vi "Module Top Level.vi"(8 "error in (no error)":errorcluster) -> (0 "error out":errorcluster)   [LabVIEW 2018, in "File IO.lvlib"]
doc: "This is the top level VI for this module. It uses a queue for communications and is stopped user a user event. The general architecture is similar to a simple queued message handler.\n\nThe VIs associated with this module are organized in a LabVIEW Library."
uses:
  File IO.lvlib
  Private Controls/File IO Data.ctl
  Controller (Host)/Public Controls/Test Information.ctl
  Controller (Host)/Public VIs/PreorPostSB.ctl
  Controller (Host)/Public Controls/APU Select.ctl
  Top Level/Shared Controls/Analyzed Data Sets.ctl
  Top Level/Shared Controls/All Data Cluster.ctl
  Top Level/Shared Controls/Acq Data.ctl
  Top Level/Shared Controls/APU Setup File.ctl
  <vilib>/Utility/NIReport.llb/NI_report.lvclass
  Private Controls/Module Data.ctl
  Private Controls/Module Action.ctl
  Public Controls/Write to Report.ctl
  Public Controls/Report Sheet Names.ctl
  <vilib>/Utility/NIReport.llb/Report Type.ctl
  Public Controls/Variables.ctl
  Testing UI 3/Public Controls/Accel Config.ctl
  Testing UI 3/Private Controls/Cutoff Frequency.ctl
  <vilib>/Utility/file.llb/Write Delimited Spreadsheet (string).vi
  Error Handler/Error Handler.lvlib
  Controller (Host)/Controller (Host).lvlib
  Testing UI 1/Testing UI 1.lvlib
  Testing UI 2/Testing UI 2.lvlib
  Testing UI 3/Testing UI 3.lvlib
  <vilib>/Utility/NIReport.llb/NI_ReportGenerationCore.lvlib
panel:
  in  "Record Data Test":bool
  in  "Test APU RUN TIME LOG":bool
  # "File I/O"
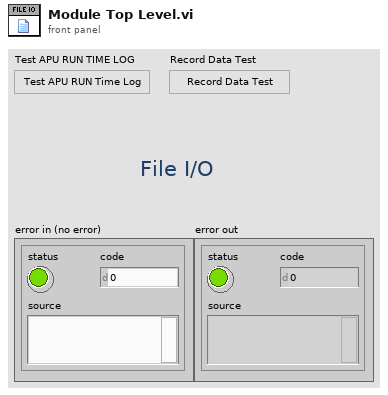
[diagram p1: front panel]
types:
  T1 = typedef "File IO.lvlib/File IO Data.ctl" = cluster{"System Log File":path, "Data File":path, "Work Order Folder":path, "Report Template Folder":path, "Report Folder":path, "Report File":path, "APU Setup Folder":path, "Testing State":bool, "Recording State":bool, "Test Information":T2, "Crash Log Data":T5, "Group Name":string, "APU Setup":T8, "ChannelTagsToLog":string[], "report ref":refnum<class "NI_report.lvclass">, "APU Setup File":path, "RunTimes":string[], "ReportHeader":string[]}
  T2 = typedef "Controller (Host).lvlib/Test Information.ctl" = cluster{"APU Part Number:":string, "Model:":string, "Serial Number:":string, "Customer:":string, "Work Order:":string, "Pre or Post SB":T3, "Run Count":i32, "APU Selected":T4}
  T3 = typedef "Controller (Host).lvlib/PreorPostSB.ctl" = string
  T4 = typedef "Controller (Host).lvlib/APU Select.ctl" = string
  T5 = typedef "Analyzed Data Sets.ctl" = T6[]
  T6 = typedef "All Data Cluster.ctl" = cluster{"AI":T7, "Accel Data":cluster{"Accel RMS(in/sec2)":dbl[], "Accel Peak(in/sec2)":dbl[], "Velocity RMS(in/sec)":dbl[], "Velocity Peak(in/sec)":dbl[]}, "Temps":cluster{"01-00-9213":dbl[], "01-01-9213":dbl[], "01-02-9213":dbl[]}, "00-03-9402(RPM)":dbl[], "02-04-9871":dbl[], "ARINC":sgl[]}
  T7 = typedef "Acq Data.ctl" = cluster{"00-00-9220":dbl[], "00-01-9220":dbl[], "02-02-9219":dbl[], "02-03-9227":dbl[], "02-05-9205":dbl[]}
  T8 = typedef "APU Setup File.ctl" = cluster{"Sensor Info":string[][], "Variables":string[][], "CMM Table 106":string[][], "CMM Table 106B ":string[][], "Accel Config":string[][], "Report Sheet 1":string[][], "Report Sheet 2":string[][], "Report Sheet 3":string[][]}
  T9 = typedef "File IO.lvlib/Write to Report.ctl" = cluster{"Sheet Name":T10, "Cell #":string, "Data":string}
  T10 = typedef "File IO.lvlib/Report Sheet Names.ctl" = string
  T11 = typedef "NI_ReportGenerationCore.lvlib/Report Type.ctl" = enum16{"HTML", "Word", "Excel"}
  T12 = enum16{"maximized", "minimized", "normal", "no change"}
  T13 = typedef "File IO.lvlib/Variables.ctl" = cluster{"AIN":dbl, "SG60":dbl, "K":dbl, "OrifDia":dbl, "FuelPressure":dbl}
  T14 = typedef "Testing UI 3.lvlib/Accel Config.ctl" = cluster{"PS Sens":dbl, "GB Sens":dbl, "FAN Sens":dbl, "PS Cutoff Frequency":T15, "GB Cutoff Frequency":T15, "Fan Cutoff Frequency":T15}
  T15 = typedef "Testing UI 3.lvlib/Cutoff Frequency.ctl" = cluster{"LP Passband":dbl, "HP Stopband":dbl, "LP Stopband":dbl, "HP Passband":dbl}
  T16 = typedef "File IO.lvlib/Module Data.ctl" = cluster{"Data":variant, "Action":T17}
  T17 = typedef "File IO.lvlib/Module Action.ctl" = enum8{"Timeout", "OpenReport", "Continue Test", "Init", "Error", "Exit", "Save Accel Data", "Set Recording State", "Log APU RunTime", "Start New Test", "Create New Reports", "Write to System Log", "Save Variables", "Load APU Setup File", "Increment Run Count", "Write To Report"}
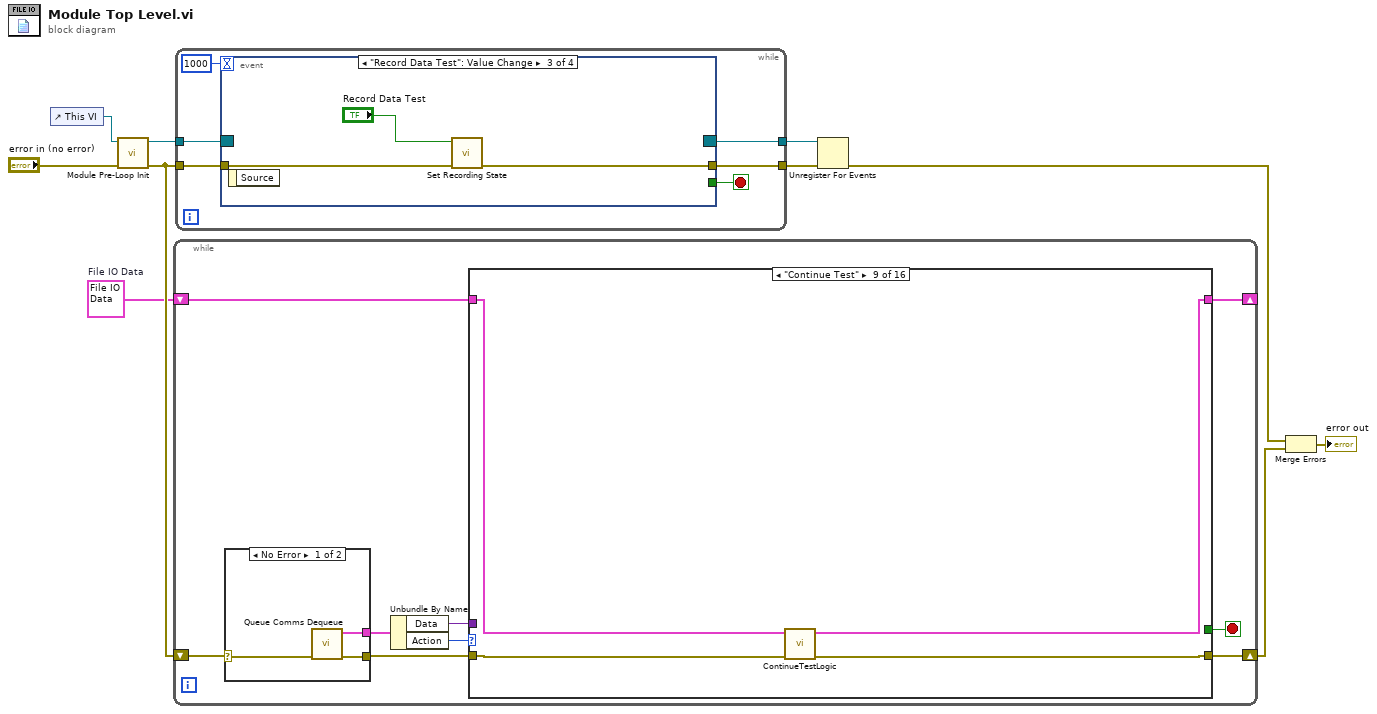
[diagram p0: block diagram]
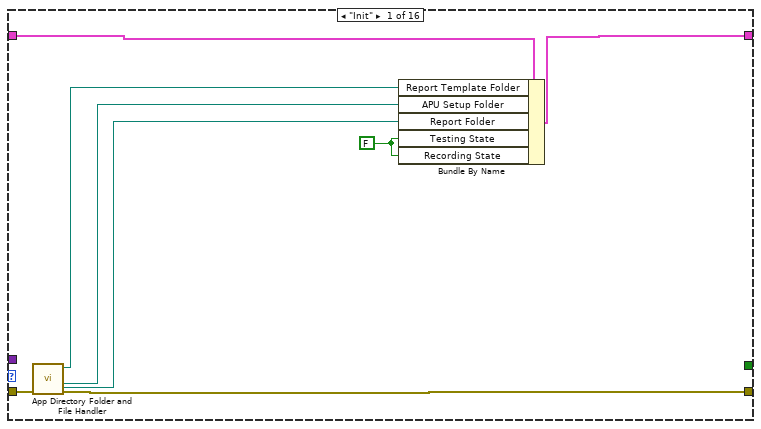
[diagram p2: hidden frame]
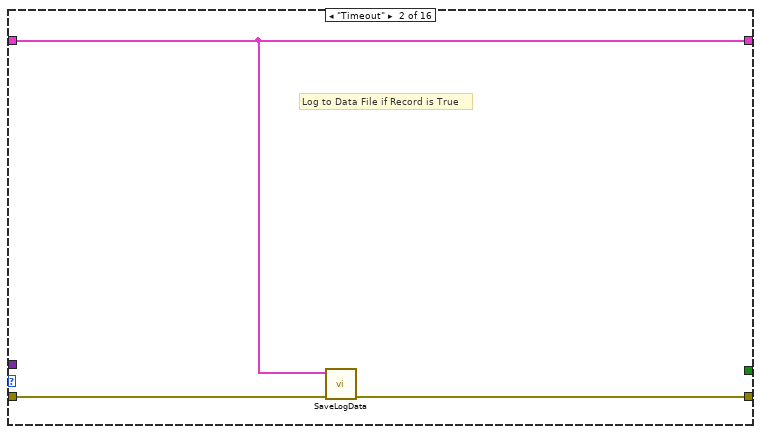
[diagram p3: hidden frame]
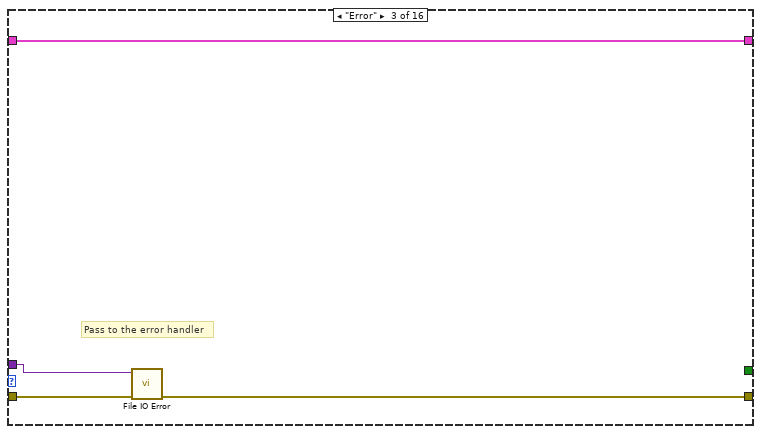
[diagram p4: hidden frame]
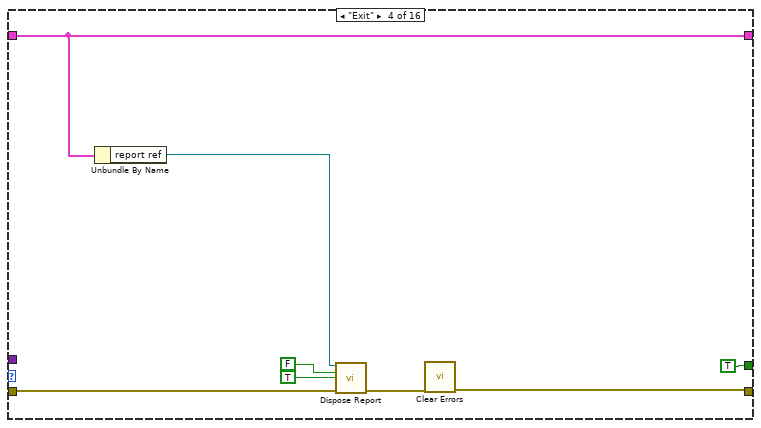
[diagram p5: hidden frame]
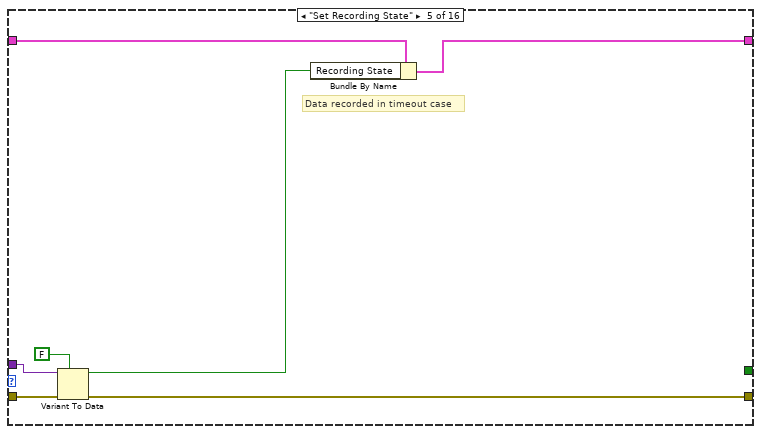
[diagram p6: hidden frame]
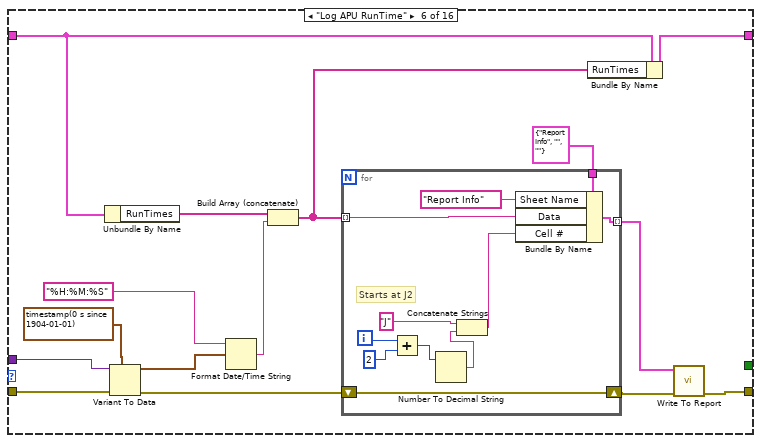
[diagram p7: hidden frame]
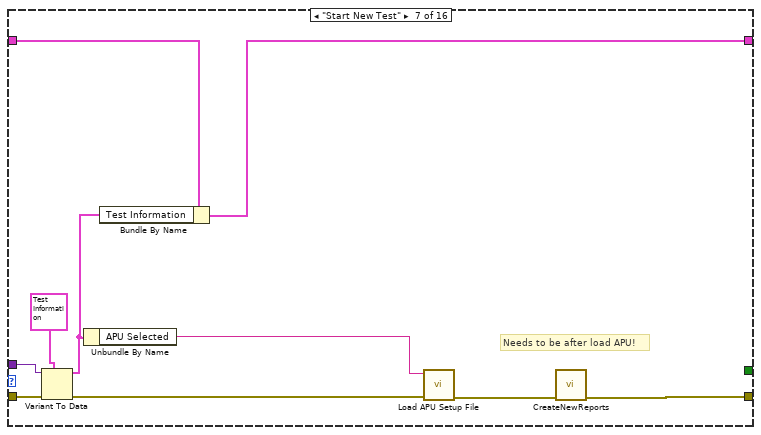
[diagram p8: hidden frame]
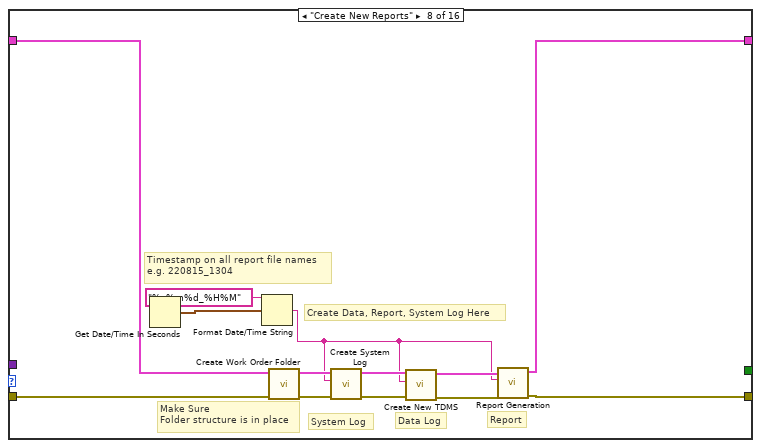
[diagram p9: hidden frame]
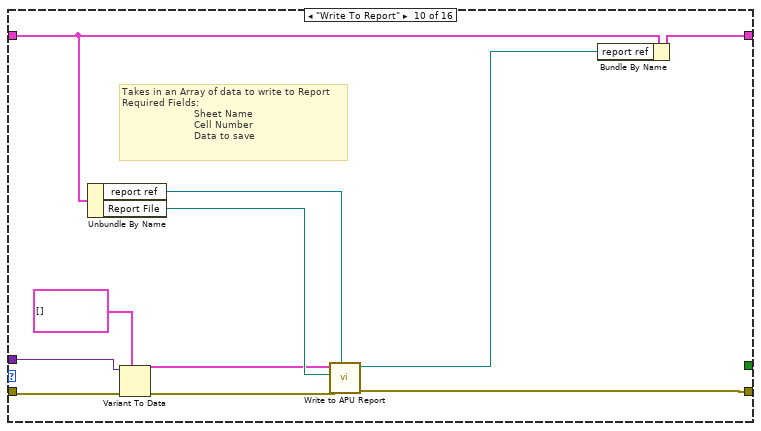
[diagram p10: hidden frame]
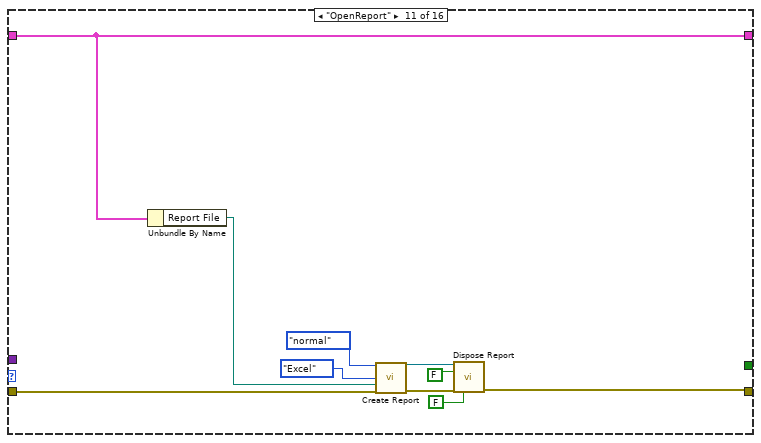
[diagram p11: hidden frame]
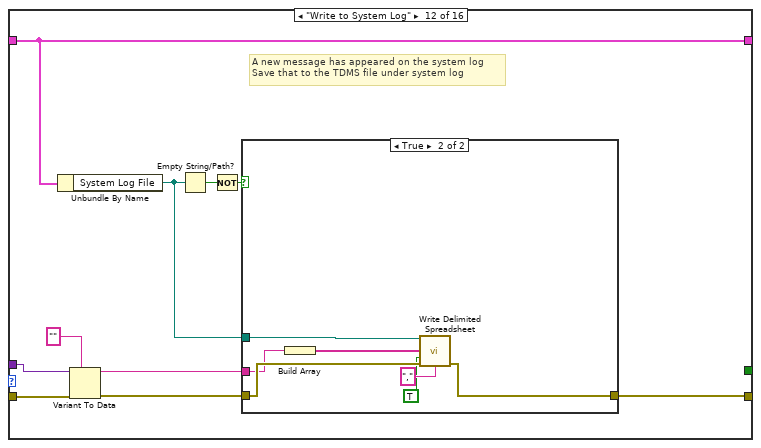
[diagram p12: hidden frame]
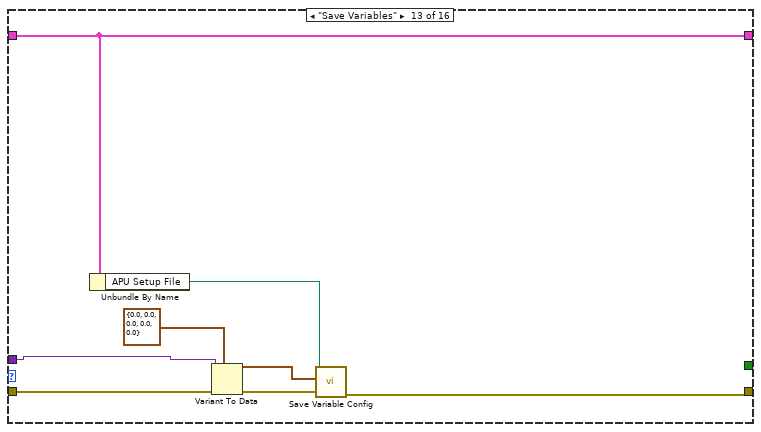
[diagram p14: hidden frame]
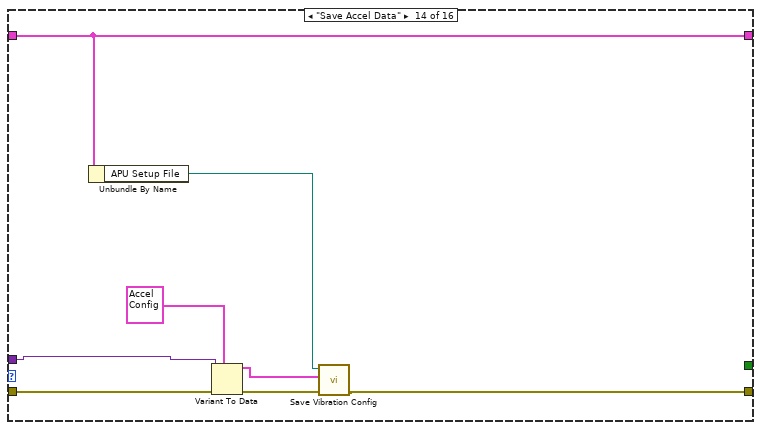
[diagram p15: hidden frame]
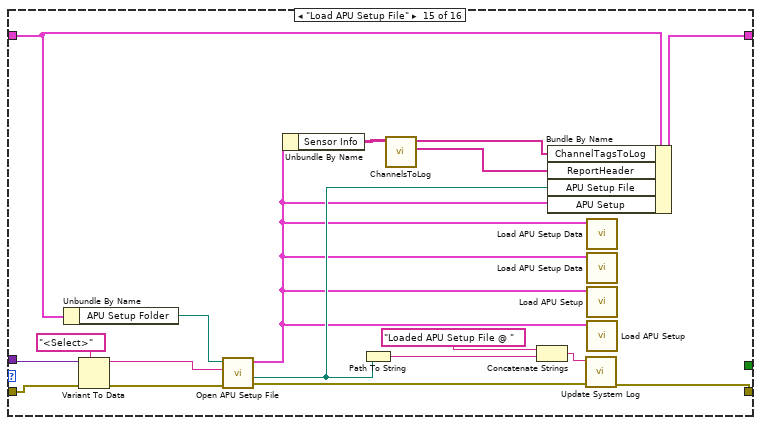
[diagram p16: hidden frame]
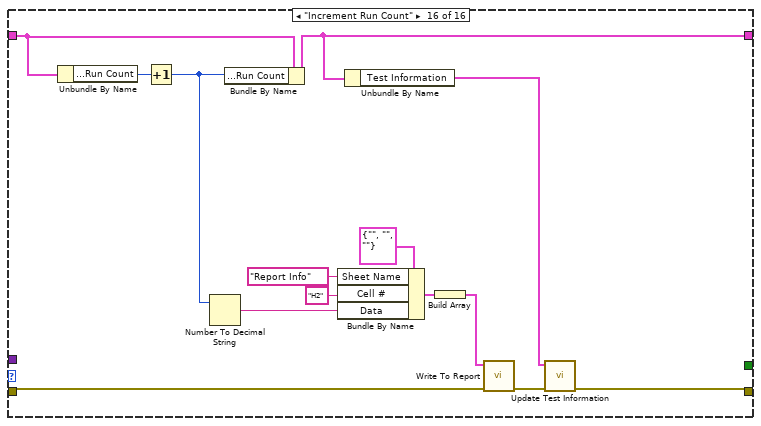
[diagram p17: hidden frame]
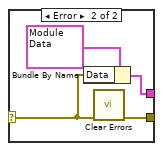
[diagram p18: hidden frame]
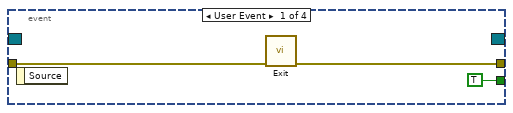
[diagram p19: hidden frame]
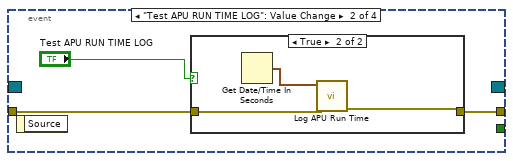
[diagram p20: hidden frame]
diagram:
  w1 = T1 {"System Log File"=path "", "Data File"=path "", "Work Order Folder"=path "", "Report Template Folder"=path "", "Report Folder"=path "", "Report File"=path "", "APU Setup Folder"=path "", "Testing State"=FALSE, "Recording State"=FALSE, "Test Information"={"APU Part Number:"="", "Model:"="", "Serial Number:"="", "Customer:"="", "Work Order:"="", "Pre or Post SB"="", "Run Count"=0, "APU Selected"="<Select>"}, "Crash Log Data"=[], "Group Name"="", "APU Setup"={"Sensor Info"=[], "Variables"=[], "CMM Table 106"=[], "CMM Table 106B "=[], "Accel Config"=[], "Report Sheet 1"=[], "Report Sheet 2"=[], "Report Sheet 3"=[]}, "ChannelTagsToLog"=[], "report ref"=refnum, "APU Setup File"=path "", "RunTimes"=[], "ReportHeader"=[]}  # File IO Data
  n1 = control-ref of="This VI"() -> (w10:refnum<vi>)
  n2 = call "Module Pre-Loop Init.vi"("error in (no error)"="error in (no error)", "Top Level VI Ref in"=w10) -> ("error out"=w4:errorcluster, "User Event Stop Ref"=w8:refnum<event-registration>)  [unwired: 8 in]
  n3 = while {
    shift-right: [w14] -> w7
    shift-left: w4 -> [w13]
    shift-right: [w11] -> _
    shift-left: w1 -> [w12]
    stop <- w15 stop-if-true
    n4 = case shown="No Error" w13 {
      selector: w13 -> [w191 w194]
      tunnel: [w192 w195] -> w19
      tunnel: [w190 w193] -> w16
      frame No Error {
        n5 = call "Queue Comms Dequeue.vi"("error in (no error)"=w191) -> ("error out"=w190:errorcluster, "element"=w192:T16)  [unwired: 9 in]
      }
      frame Error {
        n6 = Bundle By Name(cluster=T16 {"Data"=variant, "Action"=enum."Error"} ("element"), "Data"=w194) -> (w195:T16)
        n7 = call <vilib>:"Clear Errors.vi"("error in (no error)"=w194) -> ("error out"=w193:errorcluster)  [unwired: 5 in, 1 out]
      }
    }
    n8 = Unbundle By Name(w19) -> ("Data"=w17:variant, "Action"=w18:T17)
    n9 = case shown="\"Continue Test\"" w18 {
      tunnel: w17 -> [_ _ w32 _ w48 w63 w84 _ _ w108 _ w132 w148 w156 w165 _]
      tunnel: w16 -> [w27 w30 w34 w37 w49 w64 w83 w96 w99 w109 w120 w133 w149 w157 w166 w183]
      tunnel: [w20 w29 w33 w35 w43 w52 w78 w87 w100 w113 w114 w125 w144 w150 w169 w176] -> w14
      tunnel: [_ _ _ TRUE _ _ _ _ _ _ _ _ _ _ _ _] -> w15
      tunnel: w12 -> [w21 w28 w31 w41 w44 w61 w85 w94 w101 w112 w123 w130 w143 w153 w174 w189]
      tunnel: [w25 w28 w31 w41 w46 w51 w77 w86 w102 w104 w123 w130 w143 w153 w175 w179] -> w11
      frame "Init" {
        w26 = FALSE ("Testing State")
        n10 = call "App Directory Folder and File Handler.vi"("error in"=w27) -> ("error out"=w20:errorcluster, "Setup Files Folder"=w23:path, "Report Template Folder"=w24:path, "Report Folder"=w22:path)  [unwired: 7 in]
        n11 = Bundle By Name(cluster=w21, "Report Template Folder"=w24, "APU Setup Folder"=w23, "Report Folder"=w22, "Testing State"=w26, "Recording State"=w26) -> (w25:T1)
      }
      frame "Timeout" {
        # "Log to Data File if Record is True"
        n12 = call "SaveLogData.vi"("error in"=w30, "File IO Data"=w28) -> ("error out"=w29:errorcluster)  [unwired: 9 in]
      }
      frame "Error" {
        # "Pass to the error handler"
        n13 = call "File IO Error.vi"("error in (no error)"=w34, "Data"=w32) -> ("error out"=w33:errorcluster)  [unwired: 9 in]
      }
      frame "Exit" {
        n14 = Unbundle By Name(w41) -> ("report ref"=w40:refnum<class "NI_report.lvclass">)
        n15 = call-dynamic "Dispose Report.vi"("report in"=w40, "wait until printing completed? (T)"=FALSE, "save changes? (F)"=TRUE, "error in (no error)"=w37) -> ("error out"=w36:errorcluster)  [unwired: 11 in]
        n16 = call <vilib>:"Clear Errors.vi"("error in (no error)"=w36) -> ("error out"=w35:errorcluster)  [unwired: 5 in, 1 out]
      }
      frame "Set Recording State" {
        # "Data recorded in timeout case"
        n17 = Variant To Data(error in=w49, type=FALSE, Variant=w48) -> (data=w45:bool, error out=w43:errorcluster)
        n18 = Bundle By Name(cluster=w44, "Recording State"=w45) -> (w46:T1)
      }
      frame "Log APU RunTime" {
        n19 = Unbundle By Name(w61) -> ("RunTimes"=w58:string[])
        n20 = Variant To Data(error in=w64, type=timestamp(0 s since 1904-01-01) ("APU RUN TIME"), Variant=w63) -> (data=w60:timestamp, error out=w56:errorcluster)
        n21 = Format Date/Time String(time format string (%c)="%H:%M:%S", seconds (now)=w60) -> (date/time string=w57:string)  [unwired: 1 in]
        n22 = Build Array (concatenate)(w58, w57) -> (w50:string[])
        n23 = for {
          shift-right: [w75] -> w55
          shift-left: w56 -> [w75]
          tunnel: w50 -> [w74] mode=indexing
          tunnel: T9 {"Sheet Name"="Report Info", "Cell #"="", "Data"=""} ("Report Info") -> [w73]
          tunnel: [w65] -> w53 mode=indexing
          i -> [w71]
          # "Starts at J2"
          n24 = Add(x=w71, y=2) -> (x+y=w68:i32)
          n25 = Number To Decimal String(number=w68) -> (decimal integer string=w69:string)  [unwired: 1 in]
          n26 = Concatenate Strings("J", w69) -> (w66:string)
          n27 = Bundle By Name(cluster=w73, "Sheet Name"=T10 "Report Info", "Data"=w74, "Cell #"=w66) -> (w65:T9)
        }
        n28 = Bundle By Name(cluster=w61, "RunTimes"=w50) -> (w51:T1)
        n29 = call "Write To Report.vi"("error in (no error)"=w55, "Report Info"=w53) -> ("error out"=w52:errorcluster)  [unwired: 9 in]
      }
      frame "Start New Test" {
        # "Needs to be after load APU!"
        n30 = Variant To Data(error in=w83, type=T2 {"APU Part Number:"="", "Model:"="", "Serial Number:"="", "Customer:"="", "Work Order:"="", "Pre or Post SB"="", "Run Count"=0, "APU Selected"="<Select>"} ("Test Information"), Variant=w84) -> (data=w81:T2, error out=w76:errorcluster)
        n31 = Unbundle By Name(w81) -> ("APU Selected"=w80:T4)
        n32 = Bundle By Name(cluster=w85, "Test Information"=w81) -> (w77:T1)
        n33 = call "Load APU Setup File.vi"("error in (no error)"=w76, "APU Select"=w80) -> ("error out"=w79:errorcluster)  [unwired: 9 in]
        n34 = call "CreateNewReports.vi"("error in (no error)"=w79) -> ("error out"=w78:errorcluster)  [unwired: 10 in]
      }
      frame "Create New Reports" {
        # "Make Sure\nFolder structure is in place"
        # "Report"
        # "Data Log"
        # "System Log"
        # "Timestamp on all report file names\ne.g. 220815_1304"
        # "Create Data, Report, System Log Here"
        n35 = Get Date/Time In Seconds() -> (seconds since 1Jan1904=w98:timestamp)
        n36 = Format Date/Time String(time format string (%c)="%y%m%d_%H%M", seconds (now)=w98) -> (date/time string=w88:string)  [unwired: 1 in]
        n37 = call "Create Work Order Folder.vi"("error in"=w96, "File IO Data"=w94) -> ("error out"=w95:errorcluster, "File IO Data Out"=w93:T1)  [unwired: 8 in]
        n38 = call "Create System Log.vi"("error in"=w95, "TimeStamp"=w88, "File IO Data"=w93) -> ("error out"=w91:errorcluster, "File IO Data"=w92:T1)  [unwired: 7 in]
        n39 = call "Create New TDMS.vi"("error in"=w91, "TimeStamp"=w88, "File IO Data"=w92) -> ("error out"=w90:errorcluster, "File IO Data"=w89:T1)  [unwired: 7 in]
        n40 = call "Report Generation.vi"("error in"=w90, "TimeStamp"=w88, "File IO Data in"=w89) -> ("error out"=w87:errorcluster, "File IO Data out"=w86:T1)  [unwired: 7 in]
      }
      frame "Continue Test" {
        n41 = call "ContinueTestLogic.vi"("error in (no error)"=w99, "File IO Data in"=w101) -> ("error out"=w100:errorcluster, "File IO Data out"=w102:T1)  [unwired: 8 in]
      }
      frame "Write To Report" {
        # "Takes in an Array of data to write to Report\nRequired Fields:\n                        Sheet Name\n                        Cell Number\n                        Data to save"
        n42 = Unbundle By Name(w112) -> ("report ref"=w105:refnum<class "NI_report.lvclass">, "Report File"=w111:path)
        n43 = Variant To Data(error in=w109, type=T9[] [], Variant=w108) -> (data=w106:T9[], error out=w107:errorcluster)
        n44 = call "Write to APU Report.vi"("report ref"=w105, "error in"=w107, "Report Path"=w111, "data"=w106) -> ("error out"=w113:errorcluster, "report out"=w103:refnum<class "NI_report.lvclass">)  [unwired: 6 in]
        n45 = Bundle By Name(cluster=w112, "report ref"=w103) -> (w104:T1)
      }
      frame "OpenReport" {
        n46 = Unbundle By Name(w123) -> ("Report File"=w119:path)
        n47 = call <vilib>:"Create Report.vi"("window state (normal)"=T12."normal", "report type"=Report_Type."Excel", "template (empty)"=w119, "error in (no error)"=w120) -> ("report out"=w118:refnum<class "NI_report.lvclass">, "error out"=w115:errorcluster)  [unwired: 10 in]
        n48 = call-dynamic "Dispose Report.vi"("report in"=w118, "wait until printing completed? (T)"=FALSE, "error in (no error)"=w115, "close report? (T)"=FALSE) -> ("error out"=w114:errorcluster)  [unwired: 11 in]
      }
      frame "Write to System Log" {
        # "A new message has appeared on the system log\nSave that to the TDMS file under system log"
        n49 = Unbundle By Name(w130) -> ("System Log File"=w124:path)
        n50 = Variant To Data(error in=w133, type="", Variant=w132) -> (data=w128:string, error out=w129:errorcluster)
        n51 = Empty String/Path?(string/path=w124) -> (empty?=w127:bool)
        n52 = Not(x=w127) -> (.not. x?=w126:bool)
        n53 = case shown="True" w126 {
          tunnel: w129 -> [w134 w140]
          tunnel: w128 -> [_ w136]
          tunnel: [w134 w137] -> w125
          tunnel: w124 -> [_ w141]
          frame False {
            # "No System Log file yet. Start a new test or an existing test"
          }
          frame True {
            n54 = Build Array(w136) -> (w135:string[])
            n55 = call-poly <vilib>:"Write Delimited Spreadsheet.vi"("file path (dialog if empty)"=w141, "1D data"=w135, "append to file? (new file:F)"=TRUE, "error in (no error)"=w140, "delimiter (\\t)"="," ("delimiter (\\t)")) -> ("error out"=w137:errorcluster)  [unwired: 9 in, 1 out]
          }
        }
      }
      frame "Save Variables" {
        n56 = Unbundle By Name(w143) -> ("APU Setup File"=w142:path)
        n57 = Variant To Data(error in=w149, type=T13 {"AIN"=0.0, "SG60"=0.0, "K"=0.0, "OrifDia"=0.0, "FuelPressure"=0.0}, Variant=w148) -> (data=w146:T13, error out=w145:errorcluster)
        n58 = call "Save Variable Config.vi"("error in (no error)"=w145, "Variables"=w146, "Path"=w142) -> ("error out"=w144:errorcluster)  [unwired: 8 in]
      }
      frame "Save Accel Data" {
        n59 = Unbundle By Name(w153) -> ("APU Setup File"=w152:path)
        n60 = Variant To Data(error in=w157, type=T14 {"PS Sens"=0.0001, "GB Sens"=0.0001, "FAN Sens"=0.0001, "PS Cutoff Frequency"={"LP Passband"=1200.0, "HP Stopband"=250.0, "LP Stopband"=1300.0, "HP Passband"=300.0}, "GB Cutoff Frequency"={"LP Passband"=1200.0, "HP Stopband"=250.0, "LP Stopband"=1300.0, "HP Passband"=300.0}, "Fan Cutoff Frequency"={"LP Passband"=1200.0, "HP Stopband"=250.0, "LP Stopband"=1300.0, "HP Passband"=300.0}}, Variant=w156) -> (data=w151:T14, error out=w154:errorcluster)
        n61 = call "Save Vibration Config.vi"("error in (no error)"=w154, "Accell Config"=w151, "Path"=w152) -> ("error out"=w150:errorcluster)  [unwired: 8 in]
      }
      frame "Load APU Setup File" {
        n62 = Unbundle By Name(w174) -> ("APU Setup Folder"=w168:path)
        n63 = Variant To Data(error in=w166, type=T4 "<Select>" ("APU Select"), Variant=w165) -> (data=w162:T4, error out=w163:errorcluster)
        n64 = call "Open APU Setup File.vi"("error in"=w163, "APUName"=w162, "APUSetupFolder"=w168) -> ("error out"=w170:errorcluster, "APUSetupFile"=w167:path, "APU Setup File"=w161:T8)  [unwired: 6 in]
        n65 = Unbundle By Name(w161) -> ("Sensor Info"=w160:string[][])
        n66 = Path To String(path=w167) -> (string=w173:string)
        n67 = call "ChannelsToLog.vi"("Sensor Info"=w160) -> ("ReportHeader"=w158:string[], "ChannelTag"=w159:string[])  [unwired: 9 in]
        n68 = Concatenate Strings("Loaded APU Setup File @ " ("Message"), w173) -> (w171:string)
        n69 = Bundle By Name(cluster=w174, "ChannelTagsToLog"=w159, "ReportHeader"=w158, "APU Setup File"=w167, "APU Setup"=w161) -> (w175:T1)
        n70 = call "Update System Log.vi"("error in"=w170, "Message"=w171) -> ("error out"=w169:errorcluster)  [unwired: 9 in]
        n71 = call "Load APU Setup Data.vi"("APU Setup File"=w161) -> ()  [unwired: 10 in, 1 out]
        n72 = call "Load APU Setup Data.vi"("APU Setup File"=w161) -> ()  [unwired: 10 in, 1 out]
        n73 = call "Load APU Setup.vi"("APU Setup File"=w161) -> ()  [unwired: 10 in, 1 out]
        n74 = call "Load APU Setup.vi"("APU Setup File"=w161) -> ()  [unwired: 10 in, 1 out]
      }
      frame "Increment Run Count" {
        n75 = Unbundle By Name(w189) -> ("Test Information.Run Count"=w188:i32)
        n76 = Increment(x=w188) -> (x+1=w181:i32)
        n77 = Number To Decimal String(number=w181) -> (decimal integer string=w180:string)  [unwired: 1 in]
        n78 = Bundle By Name(cluster=w189, "Test Information.Run Count"=w181) -> (w179:T1)
        n79 = Bundle By Name(cluster=T9 {"Sheet Name"="", "Cell #"="", "Data"=""} ("Report Info"), "Sheet Name"=T10 "Report Info", "Cell #"="H2", "Data"=w180) -> (w184:T9)
        n80 = Unbundle By Name(w179) -> ("Test Information"=w177:T2)
        n81 = Build Array(w184) -> (w182:T9[])
        n82 = call "Write To Report.vi"("error in (no error)"=w183, "Report Info"=w182) -> ("error out"=w178:errorcluster)  [unwired: 9 in]
        n83 = call "Update Test Information.vi"("error in"=w178, "Test Information"=w177) -> ("error out"=w176:errorcluster)  [unwired: 9 in]
      }
    }
  }
  n84 = while {
    tunnel: w8 -> [w202]
    tunnel: [w201] -> w3
    tunnel: w4 -> [w200]
    tunnel: [w198] -> w2
    stop <- w199 stop-if-true
    n85 = event shown="[2] \"Record Data Test\": Value Change" {
      selector: w202 -> [_ _ _ _]
      dyn-events: [_ _ _ _] -> w198
      timeout: 1000 -> [_ _ _ _]
      tunnel: [w203 w207 w213 w216] -> w201
      tunnel: w200 -> [w204 w208 w215 w217]
      tunnel: [TRUE _ _ _] -> w199
      event User Event {
        n86 = event-data() -> ()  [unwired: 1 in, 1 out]
        n87 = call "Exit.vi"("error in"=w204) -> ("error out"=w203:errorcluster)  [unwired: 10 in]
      }
      event "Test APU RUN TIME LOG": Value Change {
        n88 = event-data() -> ()  [unwired: 1 in, 1 out]
        n89 = case shown="True" "Test APU RUN TIME LOG" {
          tunnel: w208 -> [w209 w212]
          tunnel: [w209 w211] -> w207
          frame False {
          }
          frame True {
            n90 = Get Date/Time In Seconds() -> (seconds since 1Jan1904=w210:timestamp)
            n91 = call "Log APU Run Time.vi"("error in (no error)"=w212, "APU RUN TIME"=w210) -> ("error out"=w211:errorcluster)  [unwired: 9 in]
          }
        }
      }
      event "Record Data Test": Value Change {
        n92 = event-data() -> ()  [unwired: 1 in, 1 out]
        n93 = call "Set Recording State.vi"("error in (no error)"=w215, "Recording State"="Record Data Test") -> ("error out"=w213:errorcluster)  [unwired: 9 in]
      }
      event Timeout {
        n94 = event-data() -> ()  [unwired: 1 in, 1 out]
        n95 = call "Timeout.vi"("error in (no error)"=w217) -> ("error out"=w216:errorcluster)  [unwired: 10 in]
      }
    }
  }
  n96 = Unregister For Events(event registration refnum=w2, error in=w3) -> (error out=w5:errorcluster)
  n97 = Merge Errors(w5, w7) -> (→"error out":errorcluster)
